vi "server.vi"() -> ()   [LabVIEW 2017]
uses:
  <vilib>/NI/NI JSONRPC Server Framework/Classes/Request/Request.lvclass/Request.ctl
  <vilib>/NI/NI JSONRPC Server Framework/Classes/Request/request.Read method.vi
  <vilib>/NI/NI JSONRPC Server Framework/Classes/Request/request.Read params.vi
  <vilib>/NI/NI JSONRPC Server Framework/Classes/params/params.To JSON Tree.vi
  <vilib>/NI/NI JSONRPC Server Framework/Classes/Server/Add Response (Result from Request).vi
  <vilib>/NI/NI JSONRPC Server Framework/Classes/Server/Add Response (Server Error from Request).vi
  <vilib>/NI/NI JSONRPC Server Framework/Classes/Server/Add Response (Internal Error from Request).vi
  <vilib>/NI/NI JSONRPC Server Framework/Classes/Server/Send Request (Sync).vi
  <vilib>/NI/JSON Support for LabVIEW/JSON Value/JSON Value.lvclass
  <vilib>/NI/NI JSONRPC Server Framework/Classes/Server/JSONRPC Server.lvclass
  <vilib>/NI/NI JSONRPC Server Framework/Classes/Request/Request.lvclass
panel:
  in  "stop server":bool
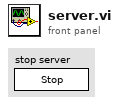
[diagram p1: front panel]
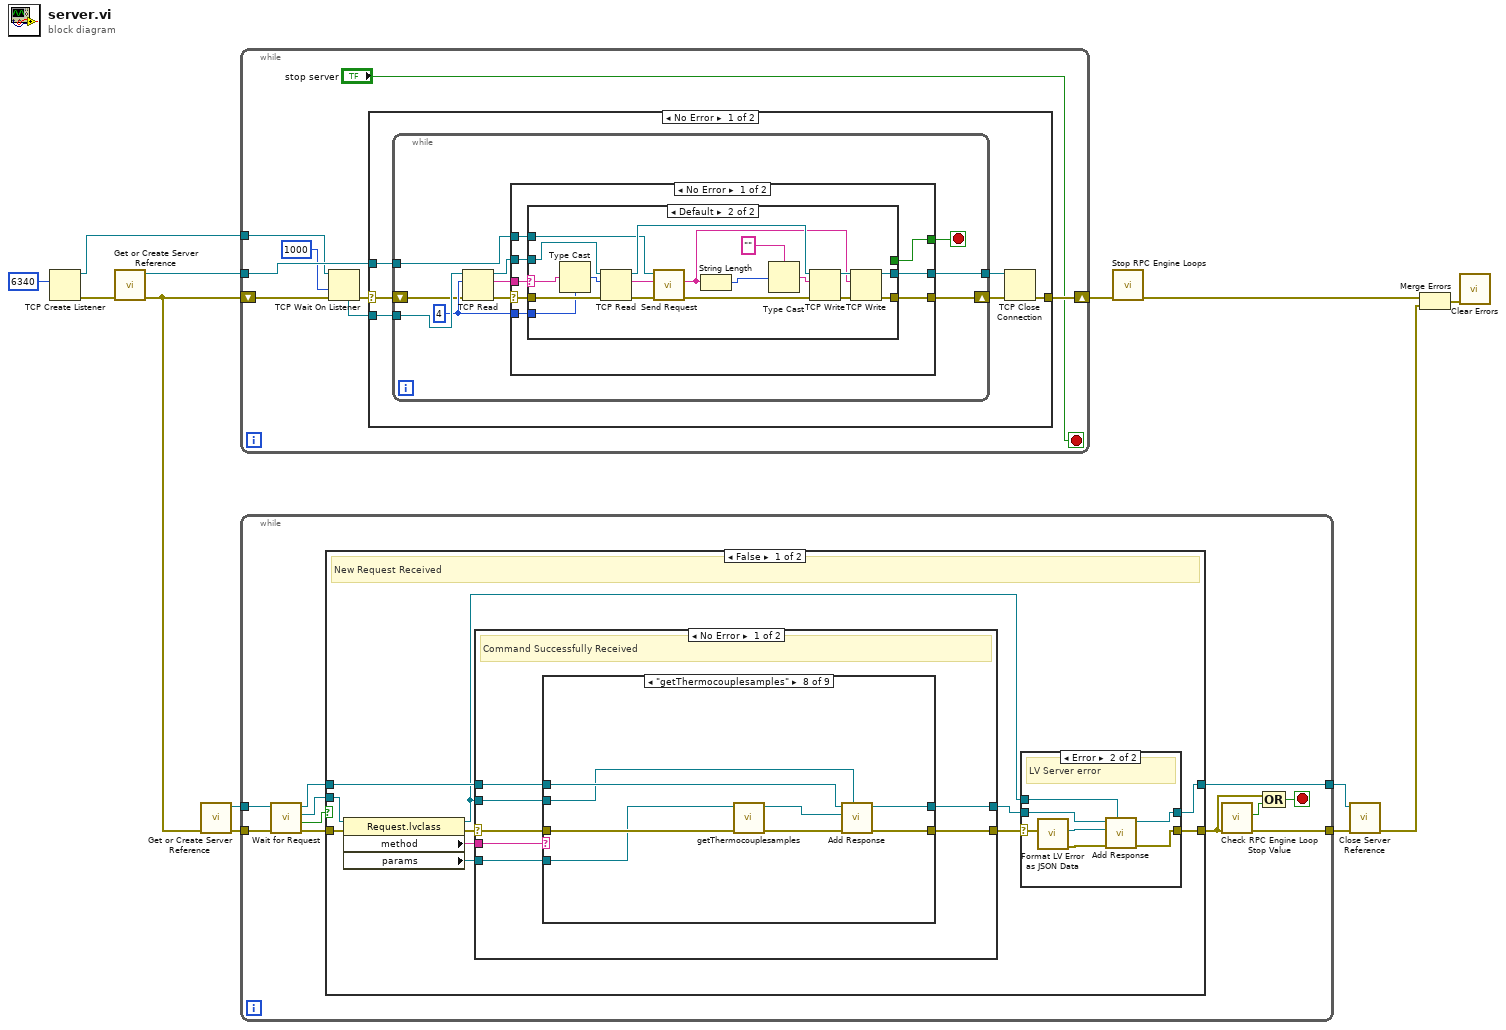
[diagram p0: block diagram]
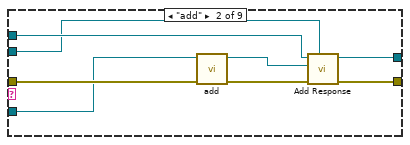
[diagram p4: hidden frame]
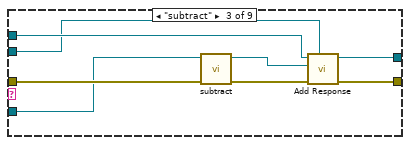
[diagram p5: hidden frame]
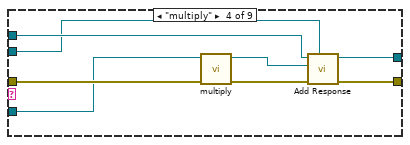
[diagram p6: hidden frame]
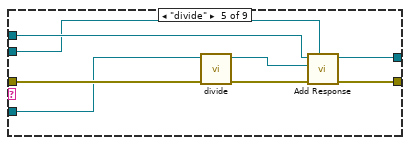
[diagram p7: hidden frame]
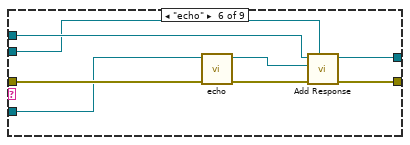
[diagram p8: hidden frame]
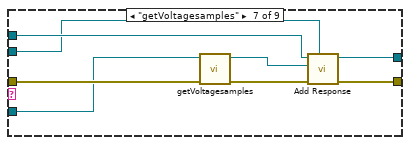
[diagram p9: hidden frame]
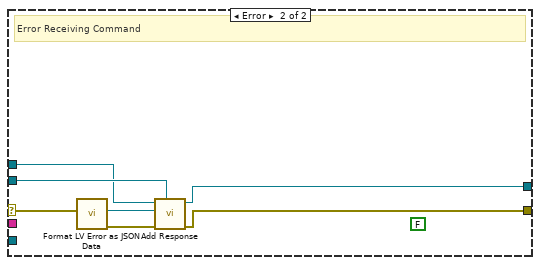
[diagram p11: hidden frame]
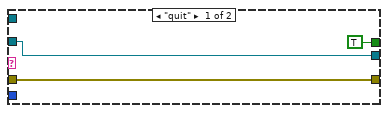
[diagram p13: hidden frame]
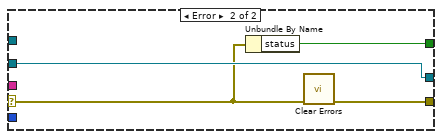
[diagram p14: hidden frame]
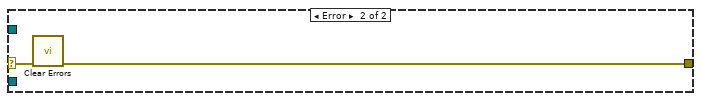
[diagram p15: hidden frame]
diagram:
  n1 = TCP Create Listener(10:u16 6340 ("remote port or service name")) -> (0:w8:errorcluster, 3:w10:refnum<k5>)  [unwired: 4 in, 1 out]
  n2 = call <vilib>:"Get or Create Server Reference.vi"("error in (no error)"=w8) -> ("error out"=w2:errorcluster, "Server Out"=w13:refnum<class "JSONRPC Server.lvclass">)  [unwired: 9 in]
  n3 = call <vilib>:"Get or Create Server Reference.vi"("error in (no error)"=w2) -> ("error out"=w4:errorcluster, "Server Out"=w3:refnum<class "JSONRPC Server.lvclass">)  [unwired: 9 in]
  n4 = while {
    tunnel: w13 -> [w21]
    tunnel: w10 -> [w19]
    shift-right: [w20] -> w12
    shift-left: w2 -> [w17]
    stop <- "stop server" stop-if-true
    n5 = TCP Wait On Listener(8:w17, 9:1000 ("timeout ms (wait forever: -1)"), 11:w19) -> (0:w16:errorcluster, 4:w18:refnum<k5>)  [unwired: 1 in, 3 out]
    n6 = case shown="No Error" w16 {
      selector: w16 -> [w22 w72]
      tunnel: w21 -> [w27 _]
      tunnel: [w26 w71] -> w20
      tunnel: w18 -> [w23 _]
      frame No Error {
        n7 = while {
          tunnel: w27 -> [w37]
          shift-right: [w29] -> w25
          shift-left: w22 -> [w30]
          tunnel: [w36] -> w24
          tunnel: w23 -> [w35]
          stop <- w28 stop-if-true
          w32 = 4 ("bytes to read")
          n8 = TCP Read(connection ID=w35, bytes to read=w32, error in (no error)=w30) -> (connection ID out=w33:refnum<k5>, data out=w34:string, error out=w31:errorcluster)  [unwired: 2 in]
          n9 = case shown="No Error" w31 {
            selector: w31 -> [w45 w68]
            tunnel: w34 -> [w44 _]
            tunnel: w33 -> [w43 w69]
            tunnel: [w42 w69] -> w36
            tunnel: [w41 w70] -> w29
            tunnel: w32 -> [w40 _]
            tunnel: w37 -> [w39 _]
            tunnel: [w38 w67] -> w28
            frame No Error {
              n10 = case shown="Default" w44 {
                selector: w44 -> [_ w65]
                tunnel: w45 -> [w48 w66]
                tunnel: w43 -> [w47 w64]
                tunnel: [w47 w63] -> w42
                tunnel: [w48 w62] -> w41
                tunnel: w40 -> [_ w54]
                tunnel: w39 -> [_ w50]
                tunnel: [TRUE _] -> w38
                frame "quit" {
                }
                frame Default {
                  n11 = Type Cast(type=w54, x=w65) -> (*(type *) &x=w55:i32)
                  n12 = TCP Read(connection ID=w64, bytes to read=w55, error in (no error)=w66) -> (connection ID out=w59:refnum<k5>, data out=w49:string, error out=w53:errorcluster)  [unwired: 2 in]
                  n13 = call-poly <vilib>:"Send Request.vi"("error in (no error)"=w53, "JSON Request String"=w49, "JSONRPC Server in"=w50) -> ("error out"=w52:errorcluster, "JSON Response String"=w51:string)  [unwired: 6 in, 1 out]
                  n14 = String Length(string=w51) -> (length=w58:i32)
                  n15 = Type Cast(type="", x=w58) -> (*(type *) &x=w56:string)
                  n16 = TCP Write(connection ID=w59, data in=w56, error in (no error)=w52) -> (connection ID out=w60:refnum<k5>, error out=w61:errorcluster)  [unwired: 1 in, 1 out]
                  n17 = TCP Write(connection ID=w60, data in=w51, error in (no error)=w61) -> (connection ID out=w63:refnum<k5>, error out=w62:errorcluster)  [unwired: 1 in, 1 out]
                }
              }
            }
            frame Error {
              n18 = Unbundle By Name(w68) -> ("status"=w67:bool)
              n19 = call <vilib>:"Clear Errors.vi"("error in (no error)"=w68) -> ("error out"=w70:errorcluster)  [unwired: 5 in, 1 out]
            }
          }
        }
        n20 = TCP Close Connection(connection ID=w24, error in (no error)=w25) -> (error out=w26:errorcluster)  [unwired: 1 in, 1 out]
      }
      frame Error {
        n21 = call <vilib>:"Clear Errors.vi"("error in (no error)"=w72) -> ("error out"=w71:errorcluster)  [unwired: 5 in, 1 out]
      }
    }
  }
  n22 = while {
    tunnel: w3 -> [w83]
    tunnel: w4 -> [w79]
    tunnel: [w74] -> w6
    tunnel: [w77] -> w5
    stop <- w76 stop-if-true
    n23 = call <vilib>:"Wait for Request.vi"("error in (no error)"=w79, "Server in"=w83) -> ("error out"=w78:errorcluster, "timed out?"=w80:bool, "Request"=w81:refnum<class "Request.lvclass">, "Server out"=w82:refnum<class "JSONRPC Server.lvclass">)  [unwired: 6 in]
    n24 = case shown="False" w80 {
      tunnel: w82 -> [w89 w178]
      tunnel: w81 -> [w94 _]
      tunnel: w78 -> [w91 w179]
      tunnel: [w87 w179] -> w75
      tunnel: [w85 w178] -> w77
      frame False {
        # "New Request Received"
        n25 = property class="Request.lvclass"(reference=w94, error in=w91) -> (reference out=w84:refnum<class "Request.lvclass">, error out=w90:errorcluster, "method"=w93:string, "params"=w92:refnum<class "JSON Value.lvclass">)
        n26 = case shown="No Error" w90 {
          selector: w90 -> [w109 w172]
          tunnel: w93 -> [w110 _]
          tunnel: w92 -> [w104 _]
          tunnel: [w107 w174] -> w88
          tunnel: w89 -> [w108 w176]
          tunnel: [w106 w175] -> w86
          tunnel: w84 -> [w105 w177]
          frame No Error {
            # "Command Successfully Received"
            n27 = case shown="\"getThermocouplesamples\"" w110 {
              tunnel: w109 -> [w112 w120 w124 w132 w140 w148 w156 w164 w170]
              tunnel: w108 -> [w111 w115 w126 w134 w142 w150 w158 w166 w169]
              tunnel: [w112 w117 w128 w136 w144 w152 w160 w168 w170] -> w107
              tunnel: [w111 w116 w127 w135 w143 w151 w159 w167 w169] -> w106
              tunnel: w105 -> [_ w113 w125 w133 w141 w149 w157 w165 _]
              tunnel: w104 -> [_ w119 w123 w129 w137 w145 w155 w163 _]
              frame Default {
              }
              frame "add" {
                n28 = call "add.vi"("error in (no error)"=w120, "params"=w119) -> ("error out"=w118:errorcluster, "data"=w114:refnum<class "JSON Value.lvclass">)  [unwired: 8 in]
                n29 = call-poly <vilib>:"Add Response.vi"("Request"=w113, "error in (no error)"=w118, "JSON Value in"=w114, "Server in"=w115) -> ("error out"=w117:errorcluster, "Server out"=w116:refnum<class "JSONRPC Server.lvclass">)  [unwired: 5 in, 1 out]
              }
              frame "subtract" {
                n30 = call "subtract.vi"("error in (no error)"=w124, "params"=w123) -> ("error out"=w121:errorcluster, "data"=w122:refnum<class "JSON Value.lvclass">)  [unwired: 8 in]
                n31 = call-poly <vilib>:"Add Response.vi"("Request"=w125, "error in (no error)"=w121, "JSON Value in"=w122, "Server in"=w126) -> ("error out"=w128:errorcluster, "Server out"=w127:refnum<class "JSONRPC Server.lvclass">)  [unwired: 5 in, 1 out]
              }
              frame "multiply" {
                n32 = call "multiply.vi"("error in (no error)"=w132, "params"=w129) -> ("error out"=w131:errorcluster, "data"=w130:refnum<class "JSON Value.lvclass">)  [unwired: 8 in]
                n33 = call-poly <vilib>:"Add Response.vi"("Request"=w133, "error in (no error)"=w131, "JSON Value in"=w130, "Server in"=w134) -> ("error out"=w136:errorcluster, "Server out"=w135:refnum<class "JSONRPC Server.lvclass">)  [unwired: 5 in, 1 out]
              }
              frame "divide" {
                n34 = call "divide.vi"("error in (no error)"=w140, "params"=w137) -> ("error out"=w139:errorcluster, "data"=w138:refnum<class "JSON Value.lvclass">)  [unwired: 8 in]
                n35 = call-poly <vilib>:"Add Response.vi"("Request"=w141, "error in (no error)"=w139, "JSON Value in"=w138, "Server in"=w142) -> ("error out"=w144:errorcluster, "Server out"=w143:refnum<class "JSONRPC Server.lvclass">)  [unwired: 5 in, 1 out]
              }
              frame "echo" {
                n36 = call "echo.vi"("error in (no error)"=w148, "params"=w145) -> ("error out"=w147:errorcluster, "data"=w146:refnum<class "JSON Value.lvclass">)  [unwired: 8 in]
                n37 = call-poly <vilib>:"Add Response.vi"("Request"=w149, "error in (no error)"=w147, "JSON Value in"=w146, "Server in"=w150) -> ("error out"=w152:errorcluster, "Server out"=w151:refnum<class "JSONRPC Server.lvclass">)  [unwired: 5 in, 1 out]
              }
              frame "getVoltagesamples" {
                n38 = call "getVoltagesamples.vi"("error in (no error)"=w156, "params"=w155) -> ("error out"=w153:errorcluster, "data"=w154:refnum<class "JSON Value.lvclass">)  [unwired: 8 in]
                n39 = call-poly <vilib>:"Add Response.vi"("Request"=w157, "error in (no error)"=w153, "JSON Value in"=w154, "Server in"=w158) -> ("error out"=w160:errorcluster, "Server out"=w159:refnum<class "JSONRPC Server.lvclass">)  [unwired: 5 in, 1 out]
              }
              frame "getThermocouplesamples" {
                n40 = call "getThermocouplesamples.vi"("error in"=w164, "params"=w163) -> ("error out"=w161:errorcluster, "data"=w162:refnum<class "JSON Value.lvclass">)  [unwired: 8 in]
                n41 = call-poly <vilib>:"Add Response.vi"("Request"=w165, "error in (no error)"=w161, "JSON Value in"=w162, "Server in"=w166) -> ("error out"=w168:errorcluster, "Server out"=w167:refnum<class "JSONRPC Server.lvclass">)  [unwired: 5 in, 1 out]
              }
              frame "shutdown_rpc_server" {
              }
            }
          }
          frame Error {
            (unwired) FALSE
            # "Error Receiving Command"
            n42 = call <vilib>:"Format LV Error as JSON Data.vi"("error in"=w172) -> ("error out"=w173:errorcluster, "Error Value out"=w171:refnum<class "JSON Value.lvclass">)  [unwired: 9 in]
            n43 = call-poly <vilib>:"Add Response.vi"("Request"=w177, "error in (no error)"=w173, "data"=w171, "Server in"=w176) -> ("error out"=w174:errorcluster, "Server out"=w175:refnum<class "JSONRPC Server.lvclass">)  [unwired: 5 in, 1 out]
          }
        }
        n44 = case shown="Error" w88 {
          selector: w88 -> [w96 w99]
          tunnel: [w96 w98] -> w87
          tunnel: w86 -> [w95 w102]
          tunnel: [w95 w101] -> w85
          tunnel: w84 -> [_ w97]
          frame No Error {
          }
          frame Error {
            # "LV Server error"
            n45 = call <vilib>:"Format LV Error as JSON Data.vi"("error in"=w99) -> ("error out"=w100:errorcluster, "Error Value out"=w103:refnum<class "JSON Value.lvclass">)  [unwired: 9 in]
            n46 = call-poly <vilib>:"Add Response.vi"("Request"=w97, "error in (no error)"=w100, "data"=w103, "Server in"=w102) -> ("error out"=w98:errorcluster, "Server out"=w101:refnum<class "JSONRPC Server.lvclass">)  [unwired: 5 in, 1 out]
          }
        }
      }
      frame True {
        # "Timeout while waiting for new Requests"
      }
    }
    n47 = call <vilib>:"Check RPC Engine Loop Stop Value.vi"("error in (no error)"=w75) -> ("error out"=w74:errorcluster, "stopped?"=w73:bool)  [unwired: 9 in]
    n48 = Compound Arithmetic op=OR(w75, w73) -> (w76:bool)
  }
  n49 = call <vilib>:"Stop RPC Engine Loops.vi"("error in (no error)"=w12) -> ("error out"=w9:errorcluster)  [unwired: 10 in]
  n50 = call <vilib>:"Close Server Reference.vi"("error in (no error)"=w6, "Server in"=w5) -> ("error out"=w1:errorcluster)  [unwired: 9 in]
  n51 = Merge Errors(w9, w1) -> (w7:errorcluster)
  n52 = call <vilib>:"Clear Errors.vi"("error in (no error)"=w7) -> ()  [unwired: 5 in, 2 out]
